vi "MDAQ_READ_Sum.vi"(8 "error in":errorcluster, 10 "Mode":enum16{"ASCII"}(ring), 11 "VISA resource name":refnum<visa-resource-name>) -> (0 "error out":errorcluster, 2 "Sum":u32, 3 "VISA resource name out":refnum<visa-resource-name>)   [LabVIEW 2021]
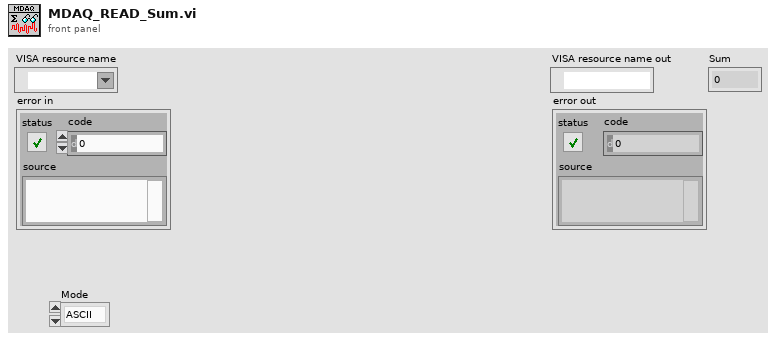
[diagram p1: front panel]
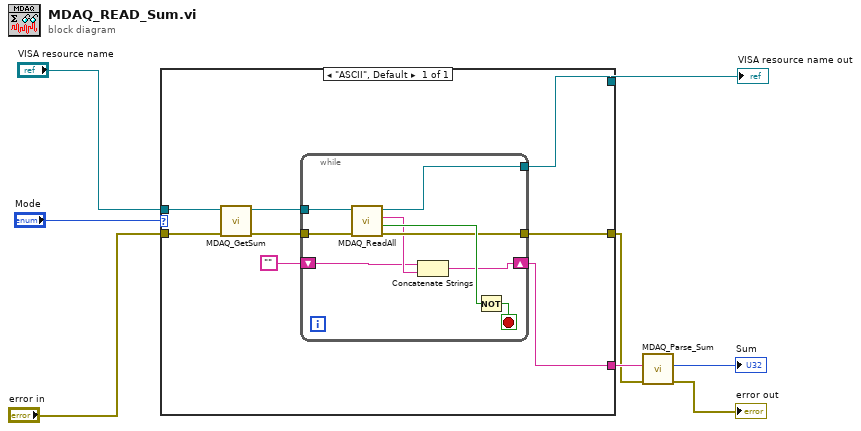
[diagram p0: block diagram]
diagram:
  n1 = case shown="\"ASCII\", Default" "Mode" {
    tunnel: "VISA resource name" -> [w12]
    tunnel: "error in" -> [w11]
    tunnel: [w16] -> w6
    tunnel: [w14] -> w4
    tunnel: [w13] -> w3
    frame "ASCII", Default {
      n2 = call "MDAQ_GetSum.vi"("error in (no error)"=w11, "VISA Refnum in"=w12) -> ("error out"=w9:errorcluster, "VISA Refnum out"=w10:refnum<visa-resource-name>)  [unwired: 8 in]
      n3 = while {
        tunnel: w10 -> [w25]
        tunnel: [w24] -> w16
        tunnel: [w21] -> w13
        shift-right: [w18] -> w14
        shift-left: "" -> [w19]
        tunnel: w9 -> [w17]
        stop <- w23 stop-if-true
        n4 = call "MDAQ_ReadAll.vi"("error in"=w17, "VISA resource name"=w25) -> ("error IO"=w21:errorcluster, "Buffer Not Empty"=w22:bool, "read buffer"=w20:string, "VISA resource name out"=w24:refnum<visa-resource-name>)  [unwired: 6 in]
        n5 = Concatenate Strings(w19, w20) -> (w18:string)
        n6 = Not(x=w22) -> (.not. x?=w23:bool)
      }
    }
  }
  "VISA resource name out" <- w6
  n7 = call "MDAQ_Parse_Sum.vi"("error in"=w3, "input buffer"=w4) -> ("error out"=→"error out":errorcluster, "Sum"=→"Sum":u32)  [unwired: 8 in]
